vi "Unregister for File Open Event.vi"(8 "error in (no error)":errorcluster, 10 "On File Open Callback":refnum<vi>, 11 "Segmented Log in":refnum<class "Segmented Log.lvclass">) -> (0 "error out":errorcluster, 3 "Segmented Log out":refnum<class "Segmented Log.lvclass">)   [LabVIEW 2015, in "Waveform Data Logger Engine.lvlib" / "Segmented Log.lvclass"]
uses:
  Segmented Log.lvclass
  Segmented Log.lvclass/Segmented Log.ctl
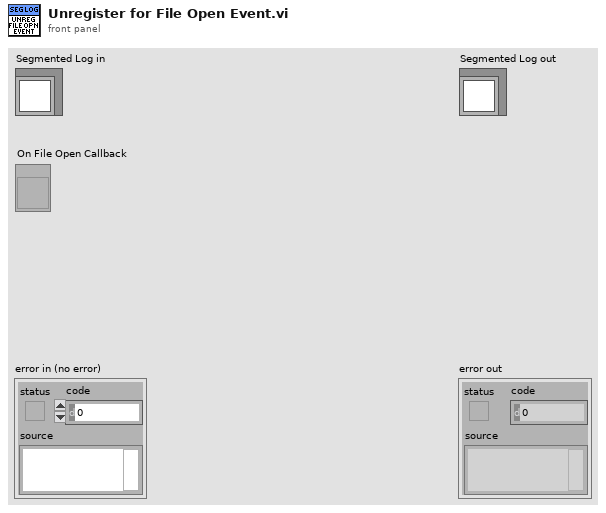
[diagram p1: front panel]
types:
  T1 = typedef "Waveform Data Logger Engine.lvlib/Segmented Log.lvclass/File Open Event Registration.ctl" = cluster{"Callback":refnum<vi>, "User Data":variant}
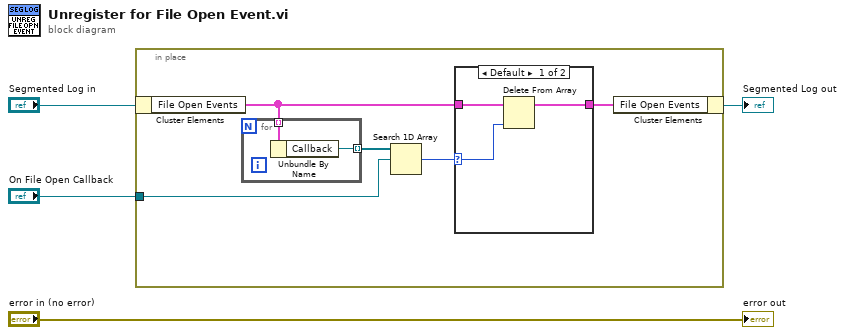
[diagram p0: block diagram]
diagram:
  n1 = in-place {
    in-place-border: "On File Open Callback" -> [w8]
    n2 = in-place-cluster #1("Segmented Log in") -> ("File Open Events"=w6:T1[])
    n3 = for {
      tunnel: w6 -> [w11] mode=indexing
      tunnel: [w10] -> w5 mode=indexing
      n4 = Unbundle By Name(w11) -> ("Callback"=w10:refnum<vi>)
    }
    n5 = Search 1D Array(1D array=w5, element=w8) -> (index of element=w7:i32)  [unwired: 1 in]
    n6 = case shown="Default" w7 {
      selector: w7 -> [w12 _]
      tunnel: [w13 w15] -> w9
      tunnel: w6 -> [w14 w15]
      frame Default {
        n7 = Delete From Array(array=w14, index=w12) -> (array with subset deleted=w13:T1[])  [unwired: 1 in, 1 out]
      }
      frame -1 {
        # "Event not registered"
      }
    }
    n8 = in-place-cluster #1("File Open Events"=w9) -> (→"Segmented Log out":refnum<class "Segmented Log.lvclass">)
  }
  "error out" <- "error in (no error)"
